vi "CSP_savePCA_Filter.vi"(8 "error in":errorcluster, 9 "File name":string="PCAFilter.bin", 11 "CSP.lvclass in":refnum<class "CSP.lvclass">) -> (0 "error out":errorcluster, 3 "CSP.lvclass out":refnum<class "CSP.lvclass">)   [LabVIEW 2016, in "Spatial Pattern Filter.lvlib" / "CSP.lvclass"]
uses:
  CSP.lvclass
  CSP.lvclass/CSP.ctl
panel:
  # "This VI is a part of BCI Design library, http://www.ru-bci.org \nCopyright © 2020, Sotnikov Peter, All rights reserved. License: GNU GPLv3"
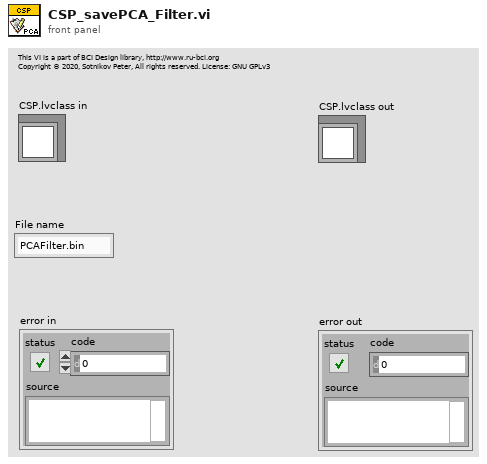
[diagram p1: front panel]
types:
  T1 = enum16{"big-endian, network order", "native, host order", "little-endian"}
  T2 = typedef "NI_Matrix.lvlib/RealMatrix.ctl" = dbl[][]
  T3 = cluster{"PCAMatrix":T2, "CovarianceMatrix":T2, "MeanValue":dbl[][]}[]
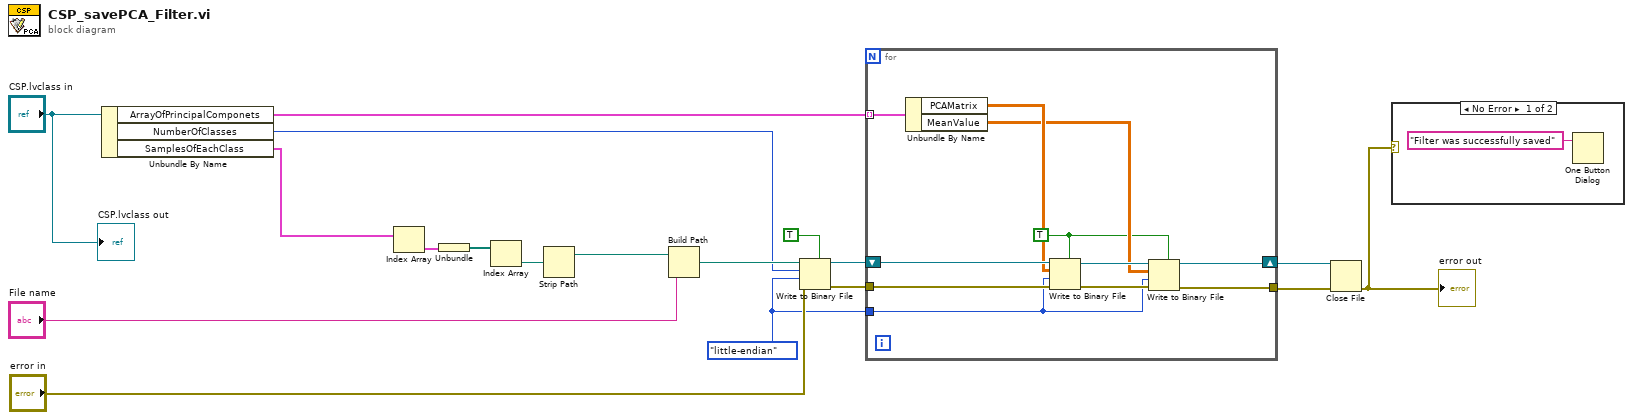
[diagram p0: block diagram]
diagram:
  w7 = T1."little-endian" ("byte order (0:big-endian, network order)")
  n1 = Unbundle By Name("CSP.lvclass in") -> ("ArrayOfPrincipalComponets"=w8:T3, "NumberOfClasses"=w12:i32, "SamplesOfEachClass"=w16:cluster{"ArrayOfFiles":path[]}[])
  n2 = Index Array(array=w16) -> (element=w3:cluster{"ArrayOfFiles":path[]})  [unwired: 1 in]
  n3 = Unbundle(w3) -> ("ArrayOfFiles"=w2:path[])
  n4 = Index Array(array=w2) -> (element=w1:path)  [unwired: 1 in]
  n5 = Strip Path(path=w1) -> (stripped path=w17:path)  [unwired: 1 out]
  n6 = Build Path(base path=w17, name or relative path="File name") -> (appended path=w14:path)
  n7 = Write to Binary File(file (use dialog)=w14, data=w12, error in="error in", 5:TRUE ("prepend array or string size? (T)"), 9:w7) -> (refnum out=w9:refnum<file>, error out=w10:errorcluster)  [unwired: 1 in, 1 out]
  n8 = for {
    tunnel: w10 -> [w28]
    tunnel: w8 -> [w29] mode=indexing
    tunnel: w7 -> [w19]
    tunnel: [w21] -> w5
    shift-right: [w20] -> w6
    shift-left: w9 -> [w27]
    w22 = TRUE ("prepend array or string size? (T)")
    n9 = Unbundle By Name(w29) -> ("PCAMatrix"=w26:T2, "MeanValue"=w23:dbl[][])
    n10 = Write to Binary File(file (use dialog)=w27, data=w26, error in=w28, 5:w22, 9:w19) -> (refnum out=w24:refnum<file>, error out=w25:errorcluster)  [unwired: 1 in, 1 out]
    n11 = Write to Binary File(file (use dialog)=w24, data=w23, error in=w25, 5:w22, 9:w19) -> (refnum out=w20:refnum<file>, error out=w21:errorcluster)  [unwired: 1 in, 1 out]
  }
  n12 = Close File(refnum=w6, error in=w5) -> (error out=w4:errorcluster)  [unwired: 1 out]
  "error out" <- w4
  n13 = case shown="No Error" w4 {
    frame No Error {
      n14 = One Button Dialog(message="Filter was successfully saved") -> ()  [unwired: 1 in, 1 out]
    }
    frame Error {
    }
  }
  "CSP.lvclass out" <- "CSP.lvclass in"
